vi "APC_9056_SensorCalibrations.vi"() -> (0 "DAQqueue":T1={"Queue array"=[0.0, 0.0, 0.0, 0.0, 0.0, 0.0, 0.0, 0.0, 0.0, 0.0, 0.0, 0.0, 0.0, 0.0, 0.0, 0.0, 0.0, 0.0, 0.0, 0.0, 0.0, 0.0, 0.0, 0.0, 0.0, 0.0, 0.0, 0.0, 0.0, 0.0, 0.0, 0.0, 0.0, 0.0, 0.0, 0.0, 0.0, 0.0, 0.0, 0.0, 0.0, 0.0, 0.0, 0.0, 0.0, 0.0, 0.0, 0.0, 0.0, 0.0, 0.0, 0.0, 0.0, 0.0, 0.0, 0.0, 0.0, 0.0, 0.0, 0.0, 0.0, 0.0, 0.0, 0.0, 0.0, 0.0, 0.0, 0.0, 0.0, 0.0, 0.0, 0.0, 0.0, 0.0, 0.0, 0.0, 0.0, 0.0, 0.0, 0.0, 0.0, 0.0, 0.0, 0.0, 0.0, 0.0, 0.0, 0.0, 0.0, 0.0, 0.0, 0.0, 0.0, 0.0, 0.0, 0.0, 0.0, 0.0, 0.0, 0.0, 0.0, 0.0, 0.0, 0.0, 0.0, 0.0, 0.0, 0.0, 0.0, 0.0, 0.0, 0.0, 0.0, 0.0, 0.0, 0.0, 0.0, 0.0, 0.0, 0.0, 0.0, 0.0, 0.0, 0.0, 0.0, 0.0, 0.0, 0.0, 0.0, 0.0, 0.0, 0.0, 0.0, 0.0, 0.0, 0.0, 0.0, 0.0, 0.0, 0.0, 0.0, 0.0, 0.0, 0.0, 0.0, 0.0, 0.0, 0.0, 0.0, 0.0, 0.0, 0.0, 0.0, 0.0, 0.0, 0.0, 0.0, 0.0, 0.0, 0.0, 0.0, 0.0, 0.0, 0.0, 0.0, 0.0, 0.0, 0.0, 0.0, 0.0, 0.0, 0.0, 0.0, 0.0], "Channel list"=["TimeStamp9056", "SystemState", "WF-TT-001", "WF-TT-002", "WF-TT-003", "WF-TT-004", "WF-TT-005", "WF-TT-006", "WF-TT-007", "WF-TT-008", "WF-TT-009", "WF-TT-010", "WF-TT-011", "WF-TT-012", "NI9220_0_12", "NI9220_0_13", "NI9220_0_14", "NI9220_0_15", "NI9208_1", "NI9208_2", "NI9208_3", "NI9208_4", "NI9220_1_4", "NI9220_1_5", "NI9220_1_6", "NI9220_1_7", "NI9220_1_8", "NI9220_1_9", "NI9220_1_10", "NI9220_1_11", "NI9220_1_12", "NI9220_1_13", "NI9220_1_14", "NI9220_1_15", "NI9214_1", "NI9214_2", "NI9214_3", "NI9214_4", "NI9214_5", "NI9214_6", "NI9214_7", "NI9214_8", "NI9214_9", "NI9214_10", "NI9214_11", "NI9214_12", "NI9214_13", "NI9214_14", "NI9214_15", "NI9214_16", "NI9264_AO0", "NI9264_AO1", "NI9264_AO2", "NI9264_AO3", "NI9264_AO4", "NI9264_AO5", "NI9264_AO6", "NI9264_AO7", "NI9264_AO8", "NI9264_AO9", "NI9264_AO10", "NI9264_AO11", "NI9264_AO12", "NI9264_AO13", "NI9264_AO14", "NI9264_AO15", "NI9375_AO0", "NI9375_AO1", "NI9375_AO2", "NI9375_AO3", "NI9375_AO4", "NI9375_AO5", "NI9375_AO6", "NI9375_AO7", "NI9375_AO8", "NI9375_AO9", "NI9375_AO10", "NI9375_AO11", "NI9375_AO12", "NI9375_AO13", "NI9375_AO14", "NI9375_AO15", "NI9266_AO0", "NI9266_AO1", "NI9266_AO2", "NI9266_AO3", "NI9266_AO4", "NI9266_AO5", "NI9266_AO6", "NI9266_AO7", "NI9375_AI0", "NI9375_AI1", "NI9375_AI2", "NI9375_AI3", "NI9375_AI4", "NI9375_AI5", "NI9375_AI6", "NI9375_AI7", "NI9375_AI8", "NI9375_AI9", "NI9375_AI10", "NI9375_AI11", "NI9375_AI12", "NI9375_AI13", "NI9375_AI14", "NI9375_AI15", "TimeStamp9049", "TimeStamp9056echo", "InjectionState", "InjEnable", "MainEnable", "MainDuration", "MainSOI", "SparkEnable", "SparkTiming", "EngineSpeed_rpm", "SystPres", "ExhaustPressure", "IMEPg1", "IMEPg2", "IMEPg3", "IMEPg4", "IMEPg5", "IMEPg6", "IMEPn1", "IMEPn2", "IMEPn3", "IMEPn4", "IMEPn5", "IMEPn6", "MaxPcyl1", "MaxPcyl2", "MaxPcyl3", "MaxPcyl4", "MaxPcyl5", "MaxPcyl6", "IMEPstd1", "IMEPstd2", "IMEPstd3", "IMEPstd4", "IMEPstd5", "IMEPstd6", "MAPO1", "MAPO2", "MAPO3", "MAPO4", "MAPO5", "MAPO6", "maxQ1", "maxQ2", "maxQ3", "maxQ4", "maxQ5", "maxQ6", "CA10_1", "CA10_2", "CA10_3", "CA10_4", "CA10_5", "CA10_6", "CA50_1", "CA50_2", "CA50_3", "CA50_4", "CA50_5", "CA50_6", "CA90_1", "CA90_2", "CA90_3", "CA90_4", "CA90_5", "CA90_6", "CylPresWarnings", "CylPresErrors"], "TS queue"=refnum, "TS signals path"="/home/lvuser/natinst/LabVIEW Data/APC_10Hz_"}, 1 "error out":errorcluster, 2 "DAQmx I tasks":refnum<k21>[](array[refnum]))   [LabVIEW 2020]
doc: "This example demonstrates the procedure required to apply different NI-DAQmx Custom Scales to each virtual channel in a task. A DAQmx Task Property Node (Functions >> NI Measurements >> DAQmx - Data Acquisition >> DAQmx Advanced Task Options) is used to obtain the task's virtual channels. A DAQmx Channel Property Node (Functions >> NI Measurements >> DAQmx - Data Acquisition) is then used to set the custom scale for each virtual channel in the task.\n\nThe \"DAQmx Create Scale\" VI creates a custom scale for each channel in the channel list. *Note, make sure your Minimum and Maximum channel parameters are consistent with the range the scale will create."
uses:
  941cde7a-e948-4dca-b3f5-25e17d4a698d.vi
  <vilib>/DAQmx/create/channels.llb/DAQmx Create Channel (AI-Current-Basic).vi
  <vilib>/DAQmx/create/channels.llb/DAQmx Create Channel (AI-Temperature-Thermocouple).vi
  <vilib>/DAQmx/configure/timing.llb/DAQmx Timing (Sample Clock).vi
  <vilib>/DAQmx/create/channels.llb/DAQmx Create Channel (AI-Voltage-Basic).vi
  <vilib>/DAQmx/create/scale.llb/DAQmx Create Scale (Linear).vi
  <resource>/objmgr/daqmx.rc
panel:
  out "DBG Chan9205":tag="Mod4/ai0:7, Mod4/ai16:23"
  out "REPEATED CHANNEL NAMES":bool
  out "WIthout replicated values":string[](array[string])=["TimeStamp9056_ms", "SystemState_i8", "WF_PT_001_bar", "WF_OA_001_O2_perc", "WF_OA_001_O2corr_perc", "WF_OA_001_Lambda_r", "WF_OA_002_O2_perc", "WF_OA_002_Lambda_r", "WF_OA_002_NOx_ppm", "EO_PT_001_bar", "TORQUE_Nm", "NI9205_9_V", "NI9205_10_V", "NI9205_11_V", "NI9205_12_V", "NI9205_13_V", "NI9205_14_V", "NI9205_15_V", "NG_FT_001_kgs", "NG_PT_001_bar", "NGDI_PT_001_bar", "O2_FC_001_kgs", "NG_FC_001_kgs", "NGDI_FT_001_kgs", "WF_PT_004_bar", "O2_PT_001_bar", "AR_PT_001_bar", "AR_FT_001_kgs", "WF_PT_016_bar", "WF_PT_014_bar", "SW_FT_001_kgs", "SW_FT_002_kgs", "SW_FT_003_kgs", "SW_FT_004_kgs", "WF_TT_001_degC", "O2_TT_001_degC", "AR_TT_001_degC", "NG_TT_001_degC", "NGDI_TT_001_degC", "WF_TT_002 _degC", "WF_TT_003_degC", "WF_TT_004_degC", "WF_TT_007_degC", "PC_TT_001_degC", "PC_TT_002_degC", "PC_TT_003_degC", "PC_TT_004_degC", "PC_TT_005_degC", "PC_TT_006_degC", "EC_TT_001_degC", "EC_TT_002_degC", "SW_TT_001_degC", "SW_TT_002_degC", "SW_TT_003_degC", "SW_TT_004_degC", "SW_TT_005_degC", "SW_TT_006_degC", "SW_TT_007_degC", "SW_TT_008_degC", "SW_TT_009_degC", "EO_TT_001_degC", "EO_TT_002_degC", "NI9214b_13_degC", "NI9214b_14_degC", "NI9214b_15_degC", "NI9214b_16_degC", "NI9264_AO0_V", "NI9264_AO1_V", "NI9264_AO2_V", "NI9264_AO3_V", "NI9264_AO4_V", "NI9264_AO5_V", "NI9264_AO6_V", "NI9264_AO7_V", "NI9264_AO8_V", "NI9264_AO9_V", "NI9264_AO10_V", "NI9264_AO11_V", "NI9264_AO12_V", "NI9264_AO13_V", "NI9264_AO14_V", "NI9264_AO15_V", "O2_FC_001_REF_mA", "AR_PC_002_REF_mA", "NG_FC_001_REF_mA", "EC_FC_001_mA", "SW_FC_004_REF_mA", "SW_FC_009_mA", "DYNO_REF_mA", "NI9266_AO7_mA", "NG_FV_001_b", "O2_PV_004_b", "AR_PV_004_b", "WF_FC_001_b", "WF_FC_002_b", "WF_FC_003_b", "NI9375_AO6_b", "NI9375_AO7_b", "NI9375_AO8_b", "NI9375_AO9_b", "NI9375_AO10_b", "NI9375_AO11_b", "NI9375_AO12_b", "NI9375_AO13_b", "NI9375_AO14_b", "NI9375_AO15_b", "NI9375_AI0_b", "NI9375_AI1_b", "NI9375_AI2_b", "NI9375_AI3_b", "NI9375_AI4_b", "NI9375_AI5_b", "NI9375_AI6_b", "NI9375_AI7_b", "NI9375_AI8_b", "NI9375_AI9_b", "NI9375_AI10_b", "NI9375_AI11_b", "NI9375_AI12_b", "NI9375_AI13_b", "NI9375_AI14_b", "NI9375_AI15_b", "AIC103_CO2_ConcTarget_ack", "AT103_CO2Conc", "PV103_PressTarget_kPa_ack", "PT103_Pressure_kPa", "PV103_VlvPosTarget_pc_ack", "PV103_VlvPos_pc_fb", "AIC201_CO2_ConcTarget_ack", "AT201_CO2Conc", "FV301_FlowTarget_kgh_ack", "FT301_Flow_kgh", "FV301_VlvPosTarget_pc_ack", "FV301_VlvPos_pc_fb", "PV300_PressTarget_kPa_ack", "PT300_Pressure_kPa", "PV300_VlvPosTarget_pc_ack", "PV300_VlvPos_pc_fb", "C101_CompSpeed_rpm", "PT104_Pressure_kPa", "PT106_Pressure_kPa", "PLC_Manual_Control", "MTR_State", "MTR_HeartBeat", "PV103_Ctrl_Mode_act", "FV301_Ctrl_Mode_act", "PV300_Ctrl_Mode_act", "MTR_Diagnostic_Status", "TimeStamp9049_ms", "TimeStamp9056echo_ms", "InjectionState_b", "InjEnable_b", "MainEnable_b", "MainDuration_ms", "MainSOI_CADBTDC", "SparkEnable_b", "SparkTiming_CADBTDC", "EngineSpeed_rpm", "WF_PT_012avg_bar", "WF_PT_005avg_bar", "IMEPg1_bar", "IMEPg2_bar", "IMEPg3_bar", "IMEPg4_bar", "IMEPg5_bar", "IMEPg6_bar", "IMEPn1_bar", "IMEPn2_bar", "IMEPn3_bar", "IMEPn4_bar", "IMEPn5_bar", "IMEPn6_bar", "PMEP1_bar", "PMEP2_bar", "PMEP3_bar", "PMEP4_bar", "PMEP5_bar", "PMEP6_bar", "MaxPcyl1_bar", "MaxPcyl2_bar", "MaxPcyl3_bar", "MaxPcyl4_bar", "MaxPcyl5_bar", "MaxPcyl6_bar", "IMEPstd1_bar", "IMEPstd2_bar", "IMEPstd3_bar", "IMEPstd4_bar", "IMEPstd5_bar", "IMEPstd6_bar", "MAPO1_bar", "MAPO2_bar", "MAPO3_bar", "MAPO4_bar", "MAPO5_bar", "MAPO6_bar", "RI1", "RI2", "RI3", "RI4", "RI5", "RI6", "maxQ1_J", "maxQ2_J", "maxQ3_J", "maxQ4_J", "maxQ5_J", "maxQ6_J", "CA03_1_CADATDC", "CA03_2_CADATDC", "CA03_3_CADATDC", "CA03_4_CADATDC", "CA03_5_CADATDC", "CA03_6_CADATDC", "CA10_1_CADATDC", "CA10_2_CADATDC", "CA10_3_CADATDC", "CA10_4_CADATDC", "CA10_5_CADATDC", "CA10_6_CADATDC", "CA50_1_CADATDC", "CA50_2_CADATDC", "CA50_3_CADATDC", "CA50_4_CADATDC", "CA50_5_CADATDC", "CA50_6_CADATDC", "CA90_1_CADATDC", "CA90_2_CADATDC", "CA90_3_CADATDC", "CA90_4_CADATDC", "CA90_5_CADATDC", "CA90_6_CADATDC", "CA97_1_CADATDC", "CA97_2_CADATDC", "CA97_3_CADATDC", "CA97_4_CADATDC", "CA97_5_CADATDC", "CA97_6_CADATDC", "CA10CA90_1_CAD", "CA10CA90_2_CAD", "CA10CA90_3_CAD", "CA10CA90_4_CAD", "CA10CA90_5_CAD", "CA10CA90_6_CAD", "maxdpdcad1_barCAD", "maxdpdcad2_barCAD", "maxdpdcad3_barCAD", "maxdpdcad4_barCAD", "maxdpdcad5_barCAD", "maxdpdcad6_barCAD", "kappa_comp1_r", "kappa_comp2_r", "kappa_comp3_r", "kappa_comp4_r", "kappa_comp5_r", "kappa_comp6_r", "kappa_exp1_r", "kappa_exp2_r", "kappa_exp3_r", "kappa_exp4_r", "kappa_exp5_r", "kappa_exp6_r", "CylPresWarnings_u64", "CylPresErrors_u64"]
  out "NI9214error":errorcluster
  out "NI9208error":errorcluster
  out "NI9205error":errorcluster
  out "Total Signals":i32=174
  out "Signals in NI9056":i32=106
  out "CHANNEL LIST":string[](array[string])=["TimeStamp9056_ms", "SystemState_i8", "WF_PT_001_bar", "WF_OA_001_O2_perc", "WF_OA_001_O2corr_perc", "WF_OA_001_Lambda_r", "WF_OA_002_O2_perc", "WF_OA_002_Lambda_r", "WF_OA_002_NOx_ppm", "EO_PT_001_bar", "TORQUE_Nm", "NI9205_9_V", "NI9205_10_V", "NI9205_11_V", "NI9205_12_V", "NI9205_13_V", "NI9205_14_V", "NI9205_15_V", "NG_FT_001_kgs", "NG_PT_001_bar", "NGDI_PT_001_bar", "O2_FC_001_kgs", "NG_FC_001_kgs", "NGDI_FT_001_kgs", "WF_PT_004_bar", "O2_PT_001_bar", "AR_PT_001_bar", "AR_FT_001_kgs", "WF_PT_016_bar", "WF_PT_014_bar", "SW_FT_001_kgs", "SW_FT_002_kgs", "SW_FT_003_kgs", "SW_FT_004_kgs", "WF_TT_001_degC", "O2_TT_001_degC", "AR_TT_001_degC", "NG_TT_001_degC", "NGDI_TT_001_degC", "WF_TT_002 _degC", "WF_TT_003_degC", "WF_TT_004_degC", "WF_TT_007_degC", "PC_TT_001_degC", "PC_TT_002_degC", "PC_TT_003_degC", "PC_TT_004_degC", "PC_TT_005_degC", "PC_TT_006_degC", "EC_TT_001_degC", "EC_TT_002_degC", "SW_TT_001_degC", "SW_TT_002_degC", "SW_TT_003_degC", "SW_TT_004_degC", "SW_TT_005_degC", "SW_TT_006_degC", "SW_TT_007_degC", "SW_TT_008_degC", "SW_TT_009_degC", "EO_TT_001_degC", "EO_TT_002_degC", "NI9214b_13_degC", "NI9214b_14_degC", "NI9214b_15_degC", "NI9214b_16_degC", "NI9264_AO0_V", "NI9264_AO1_V", "NI9264_AO2_V", "NI9264_AO3_V", "NI9264_AO4_V", "NI9264_AO5_V", "NI9264_AO6_V", "NI9264_AO7_V", "NI9264_AO8_V", "NI9264_AO9_V", "NI9264_AO10_V", "NI9264_AO11_V", "NI9264_AO12_V", "NI9264_AO13_V", "NI9264_AO14_V", "NI9264_AO15_V", "O2_FC_001_REF_mA", "AR_PC_002_REF_mA", "NG_FC_001_REF_mA", "EC_FC_001_mA", "SW_FC_004_REF_mA", "SW_FC_009_mA", "DYNO_REF_mA", "NI9266_AO7_mA", "NG_FV_001_b", "O2_PV_004_b", "AR_PV_004_b", "WF_FC_001_b", "WF_FC_002_b", "WF_FC_003_b", "NI9375_AO6_b", "NI9375_AO7_b", "NI9375_AO8_b", "NI9375_AO9_b", "NI9375_AO10_b", "NI9375_AO11_b", "NI9375_AO12_b", "NI9375_AO13_b", "NI9375_AO14_b", "NI9375_AO15_b", "NI9375_AI0_b", "NI9375_AI1_b", "NI9375_AI2_b", "NI9375_AI3_b", "NI9375_AI4_b", "NI9375_AI5_b", "NI9375_AI6_b", "NI9375_AI7_b", "NI9375_AI8_b", "NI9375_AI9_b", "NI9375_AI10_b", "NI9375_AI11_b", "NI9375_AI12_b", "NI9375_AI13_b", "NI9375_AI14_b", "NI9375_AI15_b", "AIC103_CO2_ConcTarget_ack", "AT103_CO2Conc", "PV103_PressTarget_kPa_ack", "PT103_Pressure_kPa", "PV103_VlvPosTarget_pc_ack", "PV103_VlvPos_pc_fb", "AIC201_CO2_ConcTarget_ack", "AT201_CO2Conc", "FV301_FlowTarget_kgh_ack", "FT301_Flow_kgh", "FV301_VlvPosTarget_pc_ack", "FV301_VlvPos_pc_fb", "PV300_PressTarget_kPa_ack", "PT300_Pressure_kPa", "PV300_VlvPosTarget_pc_ack", "PV300_VlvPos_pc_fb", "C101_CompSpeed_rpm", "PT104_Pressure_kPa", "PT106_Pressure_kPa", "PLC_Manual_Control", "MTR_State", "MTR_HeartBeat", "PV103_Ctrl_Mode_act", "FV301_Ctrl_Mode_act", "PV300_Ctrl_Mode_act", "MTR_Diagnostic_Status", "TimeStamp9049_ms", "TimeStamp9056echo_ms", "InjectionState_b", "InjEnable_b", "MainEnable_b", "MainDuration_ms", "MainSOI_CADBTDC", "SparkEnable_b", "SparkTiming_CADBTDC", "EngineSpeed_rpm", "WF_PT_012avg_bar", "WF_PT_005avg_bar", "IMEPg1_bar", "IMEPg2_bar", "IMEPg3_bar", "IMEPg4_bar", "IMEPg5_bar", "IMEPg6_bar", "IMEPn1_bar", "IMEPn2_bar", "IMEPn3_bar", "IMEPn4_bar", "IMEPn5_bar", "IMEPn6_bar", "PMEP1_bar", "PMEP2_bar", "PMEP3_bar", "PMEP4_bar", "PMEP5_bar", "PMEP6_bar", "MaxPcyl1_bar", "MaxPcyl2_bar", "MaxPcyl3_bar", "MaxPcyl4_bar", "MaxPcyl5_bar", "MaxPcyl6_bar", "IMEPstd1_bar", "IMEPstd2_bar", "IMEPstd3_bar", "IMEPstd4_bar", "IMEPstd5_bar", "IMEPstd6_bar", "MAPO1_bar", "MAPO2_bar", "MAPO3_bar", "MAPO4_bar", "MAPO5_bar", "MAPO6_bar", "RI1", "RI2", "RI3", "RI4", "RI5", "RI6", "maxQ1_J", "maxQ2_J", "maxQ3_J", "maxQ4_J", "maxQ5_J", "maxQ6_J", "CA03_1_CADATDC", "CA03_2_CADATDC", "CA03_3_CADATDC", "CA03_4_CADATDC", "CA03_5_CADATDC", "CA03_6_CADATDC", "CA10_1_CADATDC", "CA10_2_CADATDC", "CA10_3_CADATDC", "CA10_4_CADATDC", "CA10_5_CADATDC", "CA10_6_CADATDC", "CA50_1_CADATDC", "CA50_2_CADATDC", "CA50_3_CADATDC", "CA50_4_CADATDC", "CA50_5_CADATDC", "CA50_6_CADATDC", "CA90_1_CADATDC", "CA90_2_CADATDC", "CA90_3_CADATDC", "CA90_4_CADATDC", "CA90_5_CADATDC", "CA90_6_CADATDC", "CA97_1_CADATDC", "CA97_2_CADATDC", "CA97_3_CADATDC", "CA97_4_CADATDC", "CA97_5_CADATDC", "CA97_6_CADATDC", "CA10CA90_1_CAD", "CA10CA90_2_CAD", "CA10CA90_3_CAD", "CA10CA90_4_CAD", "CA10CA90_5_CAD", "CA10CA90_6_CAD", "maxdpdcad1_barCAD", "maxdpdcad2_barCAD", "maxdpdcad3_barCAD", "maxdpdcad4_barCAD", "maxdpdcad5_barCAD", "maxdpdcad6_barCAD", "kappa_comp1_r", "kappa_comp2_r", "kappa_comp3_r", "kappa_comp4_r", "kappa_comp5_r", "kappa_comp6_r", "kappa_exp1_r", "kappa_exp2_r", "kappa_exp3_r", "kappa_exp4_r", "kappa_exp5_r", "kappa_exp6_r", "CylPresWarnings_u64", "CylPresErrors_u64"]
  out "AdditionalTSSignalList-pre":string[](array[string])=["TimeStamp9056", "SystemState"]
  in  "Physical Channels 3":tag="Mod7/ai0:15, Mod8/ai0:15"
  out "channels 9214":string[](array[string])=["NI9214_1", "NI9214_2", "NI9214_3", "NI9214_4", "NI9214_5", "NI9214_6", "NI9214_7", "NI9214_8", "NI9214_9", "NI9214_10", "NI9214_11", "NI9214_12", "NI9214_13", "NI9214_14", "NI9214_15", "NI9214_16"]
  in  "Physical Channels 2":tag="Mod5/ai0:15"
  out "channels 9208":string[](array[string])=["NI9208_1", "NI9208_2", "NI9208_3", "NI9208_4", "NI9220_1_4", "NI9220_1_5", "NI9220_1_6", "NI9220_1_7", "NI9220_1_8", "NI9220_1_9", "NI9220_1_10", "NI9220_1_11", "NI9220_1_12", "NI9220_1_13", "NI9220_1_14", "NI9220_1_15"]
  out "AdditionalTSSignalList-post":string[](array[string])=["NI9264_AO0", "NI9264_AO1", "NI9264_AO2", "NI9264_AO3", "NI9264_AO4", "NI9264_AO5", "NI9264_AO6", "NI9264_AO7", "NI9264_AO8", "NI9264_AO9", "NI9264_AO10", "NI9264_AO11", "NI9264_AO12", "NI9264_AO13", "NI9264_AO14", "NI9264_AO15", "NI9375_AO0", "NI9375_AO1", "NI9375_AO2", "NI9375_AO3", "NI9375_AO4", "NI9375_AO5", "NI9375_AO6", "NI9375_AO7", "NI9375_AO8", "NI9375_AO9", "NI9375_AO10", "NI9375_AO11", "NI9375_AO12", "NI9375_AO13", "NI9375_AO14", "NI9375_AO15", "NI9266_AO0", "NI9266_AO1", "NI9266_AO2", "NI9266_AO3", "NI9266_AO4", "NI9266_AO5", "NI9266_AO6", "NI9266_AO7", "NI9375_AI0", "NI9375_AI1", "NI9375_AI2", "NI9375_AI3", "NI9375_AI4", "NI9375_AI5", "NI9375_AI6", "NI9375_AI7", "NI9375_AI8", "NI9375_AI9", "NI9375_AI10", "NI9375_AI11", "NI9375_AI12", "NI9375_AI13", "NI9375_AI14", "NI9375_AI15"]
  out "channels 9205":string[](array[string])=["WF-TT-001", "WF-TT-002", "WF-TT-003", "WF-TT-004", "WF-TT-005", "WF-TT-006", "WF-TT-007", "WF-TT-008", "WF-TT-009", "WF-TT-010", "WF-TT-011", "WF-TT-012", "NI9220_0_12", "NI9220_0_13", "NI9220_0_14", "NI9220_0_15"]
  in  "Physical Channels":tag="Mod4/ai0:7, Mod4/ai16:23"
  # "NI9205"
  # "ATTENTION: differential channels for NI9205 are 0-7 and 16-23"
  # "NI9208"
  # "NI9214"
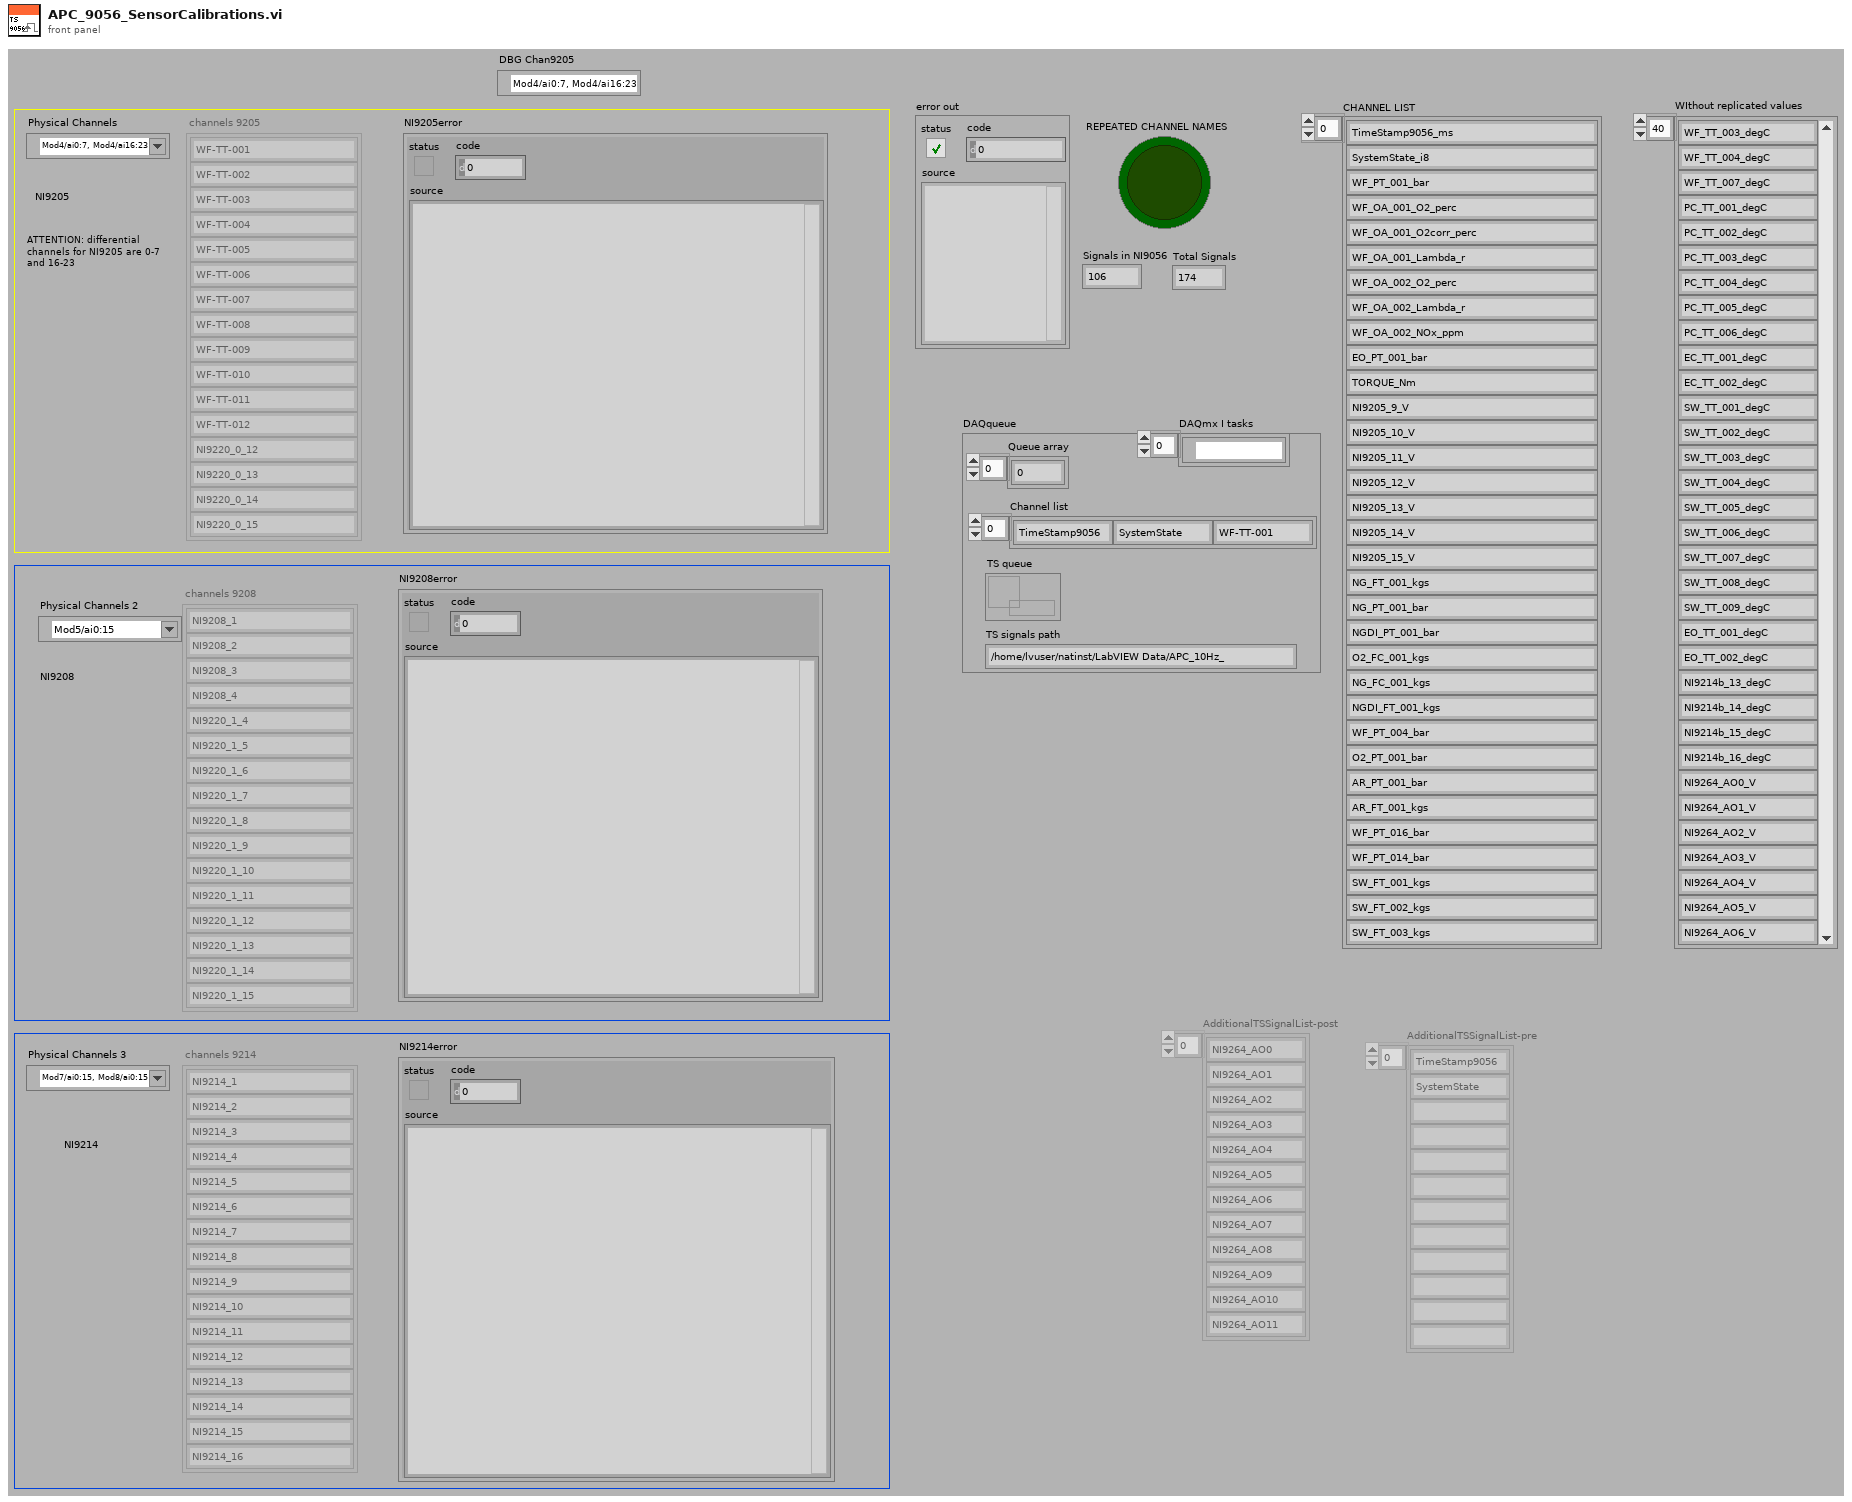
[diagram p1: front panel]
types:
  T1 = cluster{"Queue array":dbl[], "Channel list":string[], "TS queue":refnum<queue>, "TS signals path":string}
  T2 = cluster{dbl[], "result string":string[], "queue out":refnum<queue>, "TS signals path":string}
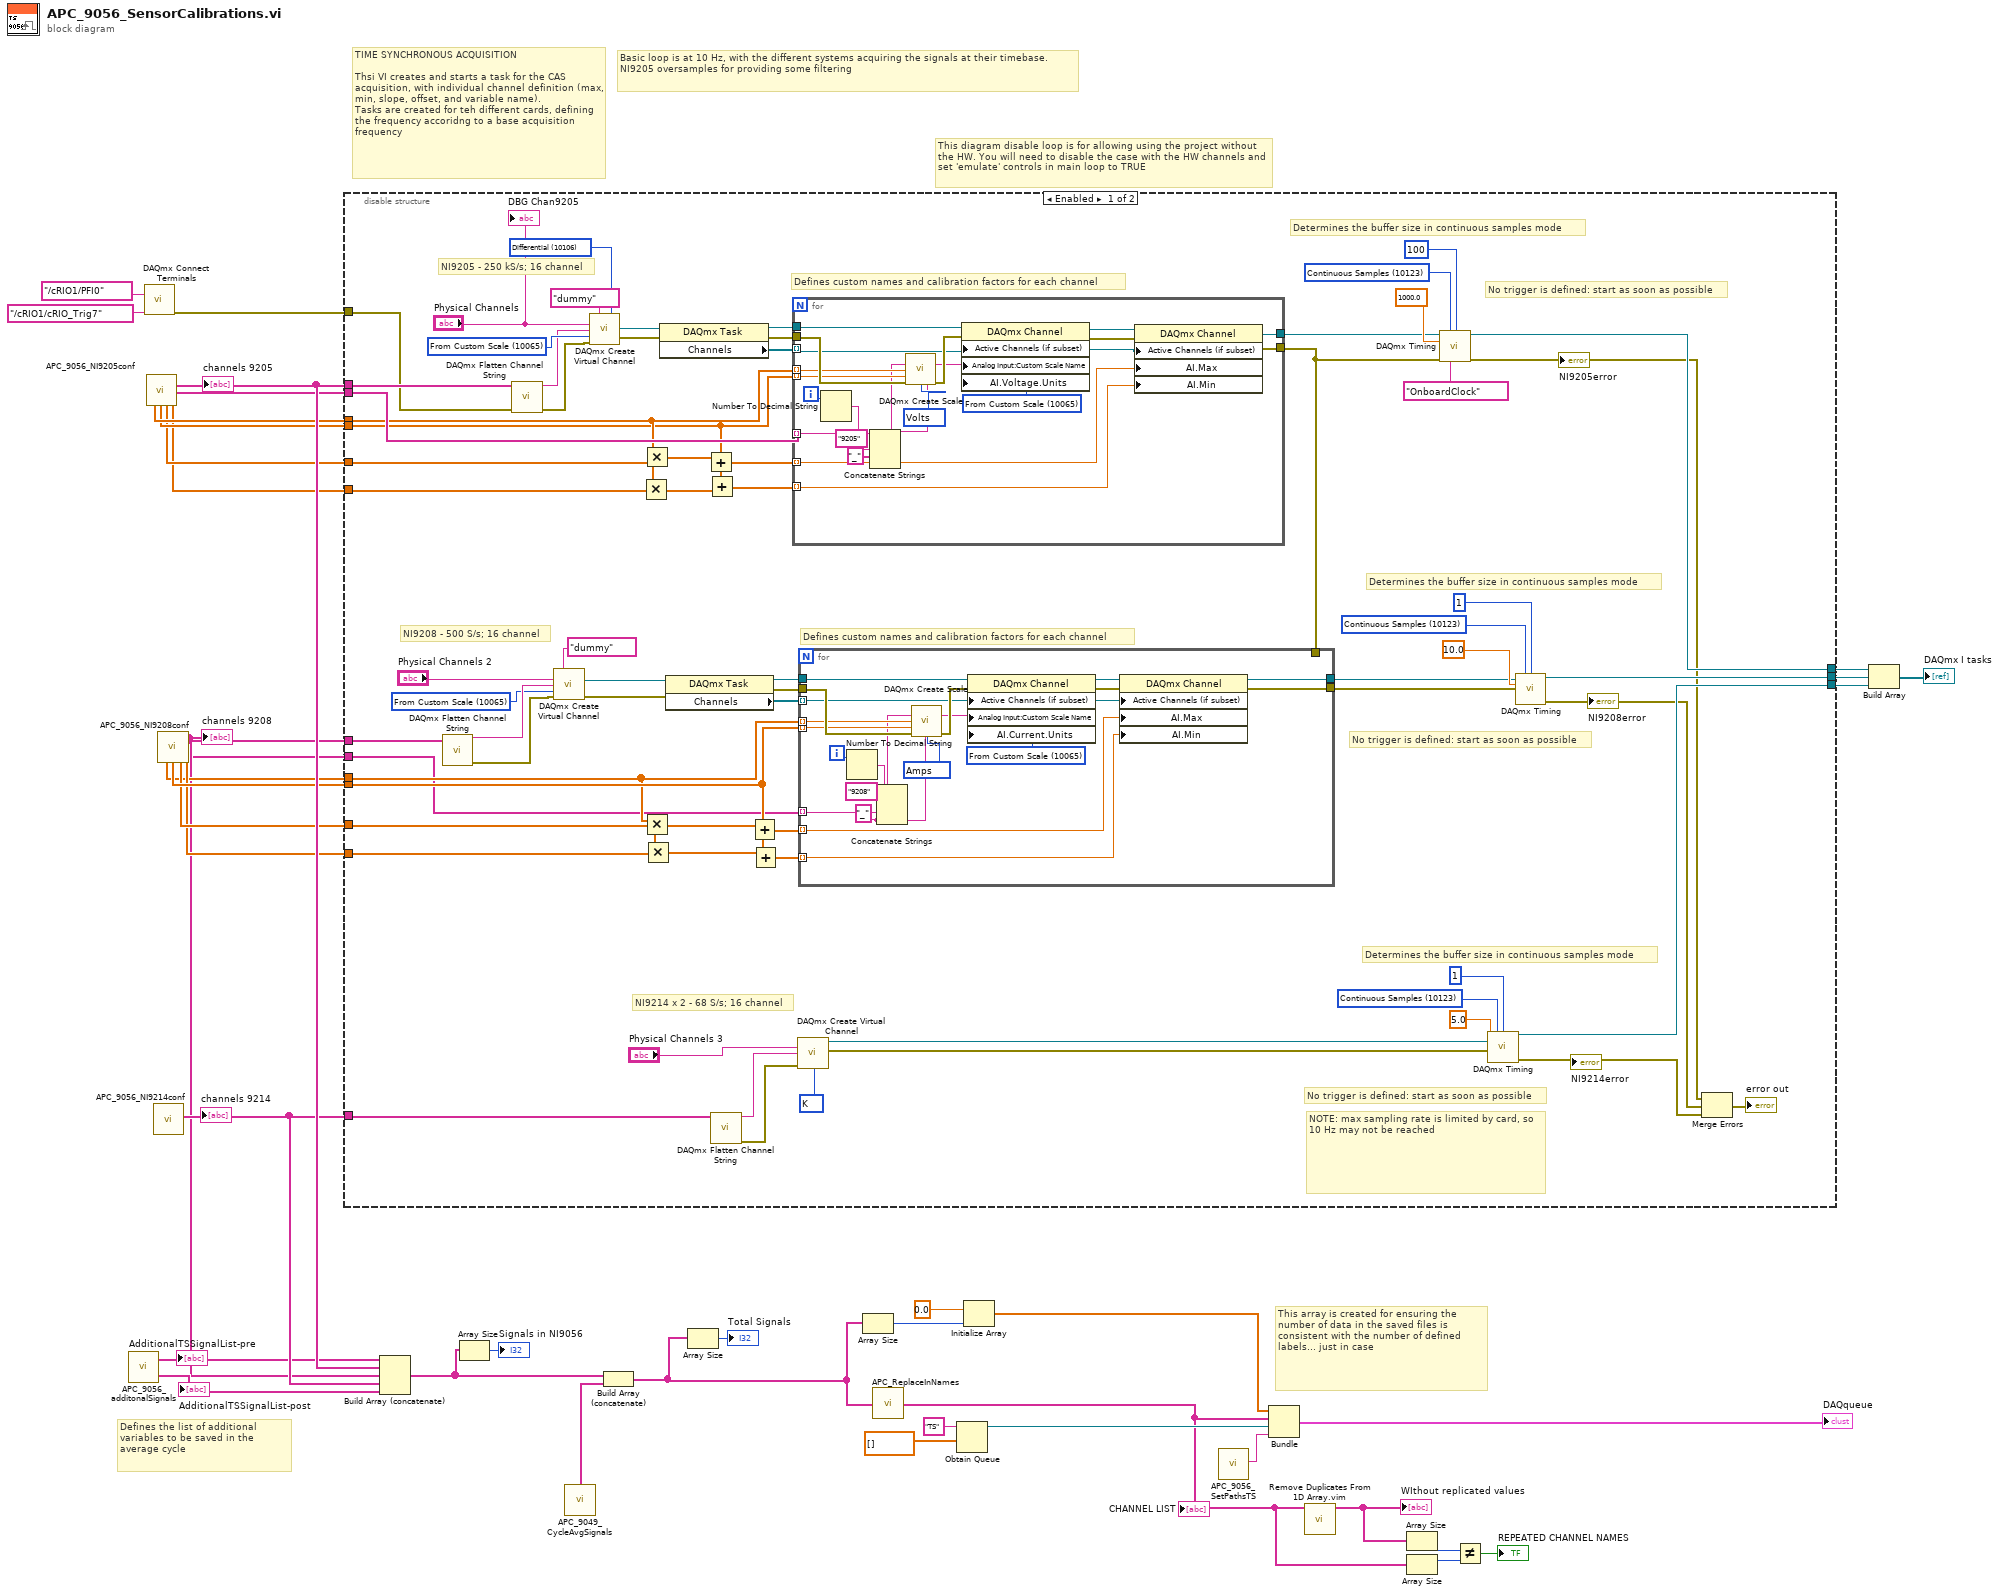
[diagram p0: block diagram]
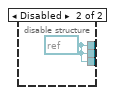
[diagram p2: hidden frame]
diagram:
  # "This diagram disable loop is for allowing using the project without the HW. You will need to disable the case with the HW channels and set 'emulate' controls in main loop to TRUE"
  # "Defines the list of additional variables to be saved in the average cycle"
  # "This array is created for ensuring the number of data in the saved files is consistent with the number of defined labels... just in case"
  # "Basic loop is at 10 Hz, with the different systems acquiring the signals at their timebase. NI9205 oversamples for providing some filtering"
  # "TIME SYNCHRONOUS ACQUISITION\n\nThsi VI creates and starts a task for the CAS acquisition, with individual channel definition (max, min, slope, offset, and variable name).\nTasks are created for teh different cards, defining the frequency accoridng to a base acquisition frequency"
  n1 = call "APC_9056_additonalSignals.vi"() -> ("AdditionalTSSignalList_post"=w22:string[], "AdditionalTSSignalList_pre"=w23:string[])  [unwired: 2 in]
  "AdditionalTSSignalList-post" <- w22
  "AdditionalTSSignalList-pre" <- w23
  n2 = call <vilib>:"DAQmx Connect Terminals.vi"("source terminal"=tag "/cRIO1/PFI0", "destination terminal"=tag "/cRIO1/cRIO_Trig7") -> ("error out"=w3:errorcluster)  [unwired: 13 in]
  n3 = call "APC_9056_NI9205conf.vi"() -> ("Min V out"=w17:dbl[], "Max V out"=w18:dbl[], "scaled units out2"=w27:string[], "Y-Intercept out"=w25:dbl[], "Slope out"=w26:dbl[], "channels name out"=w28:string[])
  "channels 9205" <- w28
  n4 = call "APC_9056_NI9214conf.vi"() -> ("channels name out"=w24:string[])  [unwired: 5 in]
  "channels 9214" <- w24
  n5 = call "APC_9056_NI9208conf.vi"() -> ("Min V out"=w5:dbl[], "Max V out"=w6:dbl[], "scaled units out2"=w1:string[], "Y-Intercept out"=w7:dbl[], "Slope out"=w4:dbl[], "channels name out"=w2:string[])
  "channels 9208" <- w2
  n6 = disable-structure shown="Enabled" {
    disable-tunnel: [w110 w153] -> w40
    disable-tunnel: [w109 w153] -> w31
    disable-tunnel: [w108 w153] -> w30
    disable-tunnel: w28 -> [w107 _]
    disable-tunnel: w27 -> [w106 _]
    disable-tunnel: w26 -> [w105 _]
    disable-tunnel: w25 -> [w104 _]
    disable-tunnel: w24 -> [w103 _]
    disable-tunnel: w18 -> [w102 _]
    disable-tunnel: w17 -> [w101 _]
    disable-tunnel: w7 -> [w100 _]
    disable-tunnel: w6 -> [w99 _]
    disable-tunnel: w5 -> [w98 _]
    disable-tunnel: w4 -> [w97 _]
    disable-tunnel: w3 -> [w96 _]
    disable-tunnel: w2 -> [w42 _]
    disable-tunnel: w1 -> [w41 _]
    frame Enabled {
      w45 = 10106 items=["Default"=-1, "RSE"=10083, "NRSE"=10078, "Differential"=10106, "Pseudodifferential"=12529] ("input terminal configuration")
      w46 = 10073 items=["J"=10072, "K"=10073, "N"=10077, "R"=10082, "S"=10085, "T"=10086, "B"=10047, "E"=10055] ("thermocouple type")
      w65 = 10123 items=["Finite Samples"=10178, "Continuous Samples"=10123, "Hardware Timed Single Point"=12522] ("sample mode")
      w75 = 10123 items=["Finite Samples"=10178, "Continuous Samples"=10123, "Hardware Timed Single Point"=12522] ("sample mode")
      w71 = 10065 items=["Volts"=10348, "From Custom Scale"=10065] ("units")
      w90 = 10123 items=["Finite Samples"=10178, "Continuous Samples"=10123, "Hardware Timed Single Point"=12522] ("sample mode")
      w94 = 10065 items=["Volts"=10348, "From Custom Scale"=10065] ("units")
      # "Defines custom names and calibration factors for each channel"
      # "NOTE: max sampling rate is limited by card, so 10 Hz may not be reached"
      # "NI9208 - 500 S/s; 16 channel"
      # "NI9214 x 2 - 68 S/s; 16 channel"
      # "No trigger is defined: start as soon as possible"
      # "Determines the buffer size in continuous samples mode"
      # "No trigger is defined: start as soon as possible"
      # "Determines the buffer size in continuous samples mode"
      # "Defines custom names and calibration factors for each channel"
      # "NI9205 - 250 kS/s; 16 channel"
      # "No trigger is defined: start as soon as possible"
      # "Determines the buffer size in continuous samples mode"
      n7 = call <vilib>:"DAQmx Flatten Channel String.vi"("names in"=w42) -> ("names out"=w72:string, "error out"=w73:errorcluster)  [unwired: 13 in]
      n8 = call <vilib>:"DAQmx Flatten Channel String.vi"("names in"=w107, "error in"=w96) -> ("names out"=w93:string, "error out"=w92:errorcluster)  [unwired: 12 in]
      n9 = call-poly <vilib>:"DAQmx Create Virtual Channel.vi"("physical channels"="Physical Channels 2", "name to assign"=w72, "units"=w71, "error in"=w73, "custom scale name"=tag "dummy") -> ("task out"=w53:refnum<k21>, "error out"=w52:errorcluster)  [unwired: 9 in]
      n10 = call-poly <vilib>:"DAQmx Create Virtual Channel.vi"("input terminal configuration"=w45, "physical channels"="Physical Channels", "name to assign"=w93, "units"=w94, "error in"=w92, "custom scale name"=tag "dummy") -> ("task out"=w80:refnum<k21>, "error out"=w79:errorcluster)  [unwired: 8 in]
      n11 = Multiply(x=w105, y=w101) -> (x*y=w82:dbl[])
      n12 = Multiply(x=w105, y=w102) -> (x*y=w83:dbl[])
      n13 = Multiply(x=w97, y=w99) -> (x*y=w56:dbl[])
      n14 = Multiply(x=w97, y=w98) -> (x*y=w55:dbl[])
      n15 = property class="DAQmx Task"(reference=w80, error in=w79) -> (reference out=w87:refnum<k21>, error out=w85:errorcluster, "Channels"=w86:refnum<k21>[])
      n16 = property class="DAQmx Task"(reference=w53, error in=w52) -> (reference out=w60:refnum<k21>, error out=w58:errorcluster, "Channels"=w59:refnum<k21>[])
      n17 = Add(x=w83, y=w104) -> (x+y=w84:dbl[])
      n18 = Add(x=w82, y=w104) -> (x+y=w81:dbl[])
      n19 = call <vilib>:"DAQmx Flatten Channel String.vi"("names in"=w103) -> ("names out"=w68:string, "error out"=w67:errorcluster)  [unwired: 13 in]
      n20 = Add(x=w56, y=w100) -> (x+y=w57:dbl[])
      n21 = Add(x=w55, y=w100) -> (x+y=w54:dbl[])
      n22 = for {
        tunnel: w87 -> [w152]
        tunnel: w86 -> [w138] mode=indexing
        tunnel: w85 -> [w151]
        tunnel: w104 -> [w147] mode=indexing
        tunnel: w106 -> [w136] mode=indexing
        tunnel: [w140] -> w78
        tunnel: [w139] -> w50
        tunnel: w84 -> [w134] mode=indexing
        tunnel: w105 -> [w146] mode=indexing
        tunnel: w81 -> [w133] mode=indexing
        i -> [w148]
        w132 = "_" ("string")
        w137 = 10065 items=["Volts"=10348, "From Custom Scale"=10065, "From TEDS"=12516] ("AI.Voltage.Units")
        w145 = 10348 items=["Volts"=10348, "From Custom Scale"=10065, "From TEDS"=12516] ("AI.Voltage.Units")
        n23 = Number To Decimal String(number=w148) -> (decimal integer string=w144:string)  [unwired: 1 in]
        n24 = Concatenate Strings("9205" ("string"), w132, w144, w132, w136) -> (w143:string)
        n25 = call-poly <vilib>:"DAQmx Create Scale.vi"("name"=w143, "slope"=w146, "y-intercept"=w147, "error in"=w151, "pre-scaled units"=w145, "scaled units"=w136) -> ("scale out"=w149:tag, "error out"=w150:errorcluster)  [unwired: 8 in]
        n26 = property class="DAQmx Channel"(reference=w152, error in=w150, "Active Channels (if subset)"=w138, "Analog Input:Custom Scale Name"=w149, "AI.Voltage.Units"=w137) -> (reference out=w142:refnum<k21>, error out=w141:errorcluster)
        n27 = property class="DAQmx Channel"(reference=w142, error in=w141, "Active Channels (if subset)"=w138, "AI.Max"=w134, "AI.Min"=w133) -> (reference out=w140:refnum<k21>, error out=w139:errorcluster)
      }
      n28 = call-poly <vilib>:"DAQmx Create Virtual Channel.vi"("physical channels"="Physical Channels 3", "name to assign"=w68, "error in"=w67, "thermocouple type"=w46) -> ("task out"=w44:refnum<k21>, "error out"=w43:errorcluster)  [unwired: 10 in]
      n29 = for {
        tunnel: w60 -> [w131]
        tunnel: w59 -> [w122] mode=indexing
        tunnel: w58 -> [w130]
        tunnel: w100 -> [w121] mode=indexing
        tunnel: w41 -> [w115] mode=indexing
        tunnel: [w126] -> w51
        tunnel: [w125] -> w49
        tunnel: w57 -> [w112] mode=indexing
        tunnel: w97 -> [w120] mode=indexing
        tunnel: w54 -> [w111] mode=indexing
        tunnel: w50 -> [_]
        i -> [w127]
        w114 = "_" ("string")
        w116 = 10065 items=["Amps"=10342, "From Custom Scale"=10065, "From TEDS"=12516] ("AI.Current.Units")
        w119 = 10342 items=["Amps"=10342, "From Custom Scale"=10065, "From TEDS"=12516] ("AI.Current.Units")
        n30 = Number To Decimal String(number=w127) -> (decimal integer string=w118:string)  [unwired: 1 in]
        n31 = Concatenate Strings("9208" ("string"), w114, w118, w114, w115) -> (w117:string)
        n32 = call-poly <vilib>:"DAQmx Create Scale.vi"("name"=w117, "slope"=w120, "y-intercept"=w121, "error in"=w130, "pre-scaled units"=w119, "scaled units"=w115) -> ("scale out"=w128:tag, "error out"=w129:errorcluster)  [unwired: 8 in]
        n33 = property class="DAQmx Channel"(reference=w131, error in=w129, "Active Channels (if subset)"=w122, "Analog Input:Custom Scale Name"=w128, "AI.Current.Units"=w116) -> (reference out=w124:refnum<k21>, error out=w123:errorcluster)
        n34 = property class="DAQmx Channel"(reference=w124, error in=w123, "Active Channels (if subset)"=w122, "AI.Max"=w112, "AI.Min"=w111) -> (reference out=w126:refnum<k21>, error out=w125:errorcluster)
      }
      n35 = call-poly <vilib>:"DAQmx Timing.vi"("task/channels in"=w78, "sample mode"=w90, "samples per channel"=100 ("number of samples per channel"), "rate"=1000.0, "source"=tag "OnboardClock", "error in"=w50) -> ("task out"=w110:refnum<k21>, "error out"=w88:errorcluster)  [unwired: 8 in]
      "NI9205error" <- w88
      n36 = call-poly <vilib>:"DAQmx Timing.vi"("task/channels in"=w44, "sample mode"=w65, "samples per channel"=1 ("number of samples per channel"), "rate"=5.0, "error in"=w43) -> ("task out"=w108:refnum<k21>, "error out"=w63:errorcluster)  [unwired: 9 in]
      "NI9214error" <- w63
      n37 = call-poly <vilib>:"DAQmx Timing.vi"("task/channels in"=w51, "sample mode"=w75, "samples per channel"=1 ("number of samples per channel"), "rate"=10.0, "error in"=w49) -> ("task out"=w109:refnum<k21>, "error out"=w62:errorcluster)  [unwired: 9 in]
      "NI9208error" <- w62
      n38 = Merge Errors(w88, w62, w63) -> (→"error out":errorcluster)
      "DBG Chan9205" <- "Physical Channels"
    }
    frame Disabled {
      w153 = refnum<k21> refnum ("task out")
    }
  }
  n39 = Build Array (concatenate)(w23, w28, w2, w24, w22) -> (w16:string[])
  n40 = Array Size(array=w16) -> (size(s)=→"Signals in NI9056":i32)
  n41 = call "APC_9049_CycleAvgSignals.vi"() -> ("CRIo9049_CycleAvgSignals"=w21:string[])  [unwired: 3 in]
  n42 = Build Array (concatenate)(w16, w21) -> (w9:string[])
  n43 = Array Size(array=w9) -> (size(s)=→"Total Signals":i32)
  n44 = Array Size(array=w9) -> (size(s)=w37:i32)
  n45 = call "APC_ReplaceInNames.vi"("string"=w9) -> ("result string"=w8:string[])
  "CHANNEL LIST" <- w8
  n46 = Obtain Queue(name (unnamed)="TS", element data type=dbl[] [] ("appended array")) -> (queue out=w35:refnum<queue>)  [unwired: 3 in, 2 out]
  n47 = Initialize Array(0.0 ("element"), w37) -> (w33:dbl[])
  n48 = call "APC_9056_SetPathsTS.vi"() -> ("TS signals path"=w34:string)  [unwired: 1 in, 2 out]
  n49 = Bundle(w33, "result string"=w8, "queue out"=w35, "TS signals path"=w34) -> (→"DAQqueue":T2)  [unwired: 1 in]
  n50 = call "Remove Duplicates From 1D Array.vim"("array"=w8) -> ("array with duplicates removed"=w13:string[])  [unwired: 10 in]
  "WIthout replicated values" <- w13
  n51 = Array Size(array=w13) -> (size(s)=w12:i32)
  n52 = Array Size(array=w8) -> (size(s)=w11:i32)
  n53 = Not Equal?(x=w12, y=w11) -> (x != y?=→"REPEATED CHANNEL NAMES":bool)
  n54 = Build Array(w40, w31, w30) -> (→"DAQmx I tasks":refnum<k21>[])
